vi "Insert Subroutine.vi"(0 "Test Executive in":refnum<class "Test Executive.lvclass">, 1 "Parent ID":string, 5 "Name":string, 9 "File Path":string, 11 "error in (no error)":errorcluster, 12 "Insertion Index":i32=-1, 13 "Path Builder":refnum<class "IPath Builder.lvclass">, 14 "Persistence":refnum<class "IPersist.lvclass">) -> (3 "Unique ID out":string, 4 "Test Executive out":refnum<class "Test Executive.lvclass">, 8 "Replaced?":bool, 15 "error out":errorcluster)   [LabVIEW 2017, in "Test Executive.lvlib" / "Test Executive.lvclass"]
uses:
  <vilib>/gpm_packages/@cs/test-executive/Source/Test Executive/TestExecutive/Test Executive.lvclass
  <vilib>/gpm_packages/@cs/persistence/source/IPersist/IPersist.lvclass
  <vilib>/gpm_packages/@cs/test-executive/Source/Path Builder/IPath Builder/IPath Builder.lvclass
  <vilib>/gpm_packages/@cs/test-executive/Source/Test Executive/Subroutine/Subroutine.lvclass
  <vilib>/gpm_packages/@cs/test-executive/Source/Test Executive/ITestExecutive/ITest Executive.lvclass
  <vilib>/gpm_packages/@cs/test-executive/Source/Test Executive/TestExecutive/Test Executive.lvclass/Test Executive.ctl
  a8f02847-2917-4e0b-9d44-6197dbaaebf7.vi
  ebcf7762-3f7b-48fa-b982-768c2ca258a4.vi
  5e1c43a7-4245-4c3f-80d4-4215ac2c26a8.vi
  5644fd4f-c316-495c-8a03-d45352207638.vi
  1c60c4bb-efd1-4132-9f22-2f49f2b93ccb.vi
  1d71063b-7a03-4771-aede-29323b453e1f.vi
  81d5cec1-e37c-4be8-84f4-52b71e3ef4cd.vi
  972ceb2e-96f1-4f86-b8d7-f01f08263765.vi
  <vilib>/gpm_packages/@cs/linked-list/Source/Linked List/ILinkedList/ILinked List.lvclass
  <vilib>/gpm_packages/@cs/linked-list/Source/Linked List/Linked List Ref/Linked List Ref.lvclass
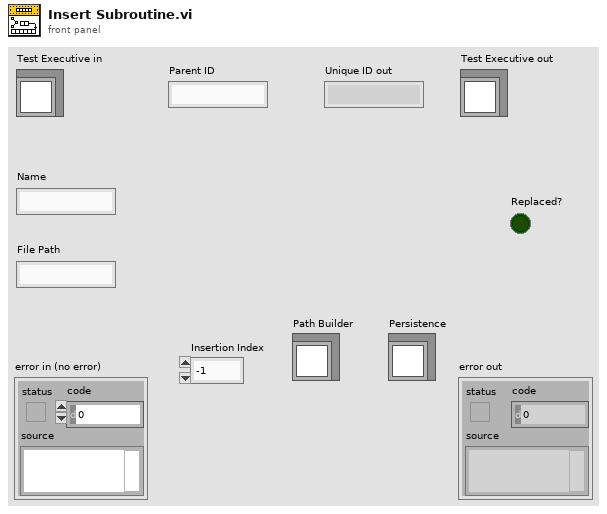
[diagram p1: front panel]
types:
  T1 = enum16{"open", "replace", "create", "open or create", "replace or create", "replace or create with confirmation"}
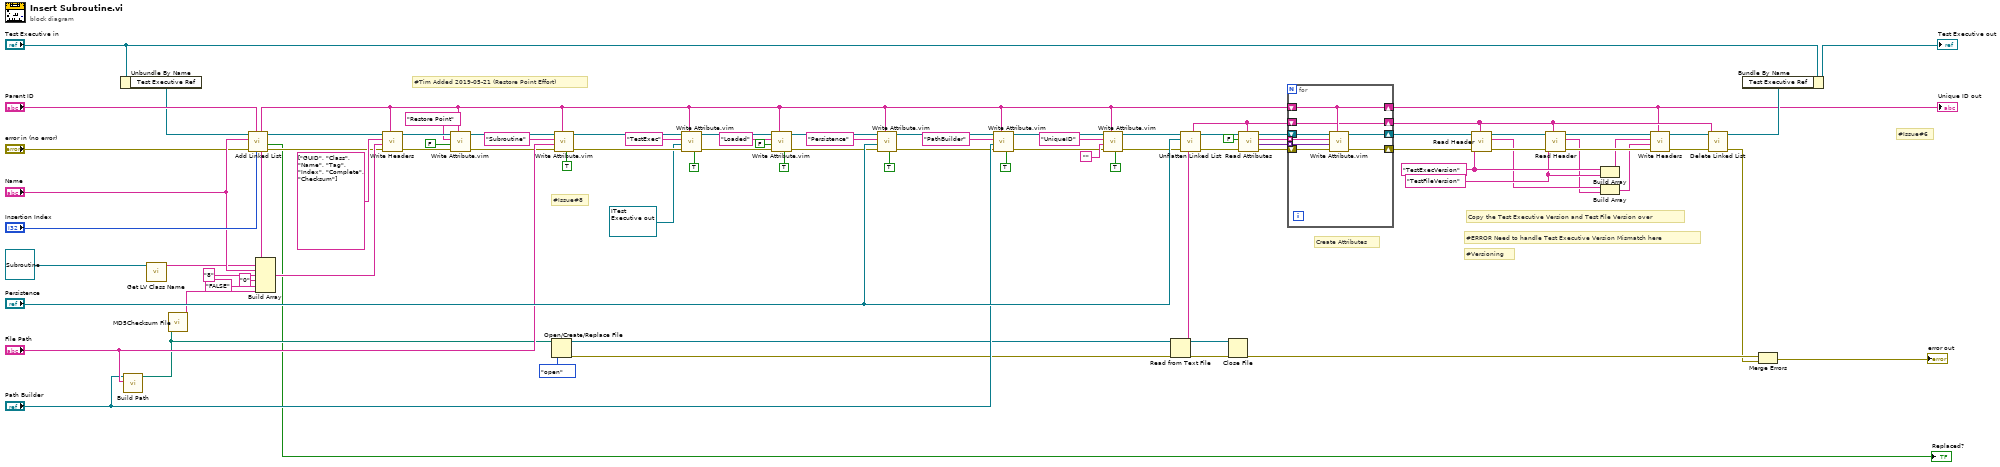
[diagram p0: block diagram]
diagram:
  w7 = "TestFileVersion" ("Header Name")
  w8 = "TestExecVersion" ("Header Name")
  # "#Versioning"
  # "#ERROR Need to handle Test Executive Version Mismatch here"
  # "Copy the Test Executive Version and Test File Version over"
  # "Create Attributes"
  # "#Issue#8"
  # "#Tim Added 2019-05-21 (Restore Point Effort)"
  # "#Issue#6"
  n1 = Unbundle By Name("Test Executive in") -> ("Test Executive Ref"=w27:refnum<data-value>)
  n2 = call-dynamic "Build Path.vi"("Path"="File Path", "IPath Builder in"="Path Builder") -> ("Path"=w26:path)  [unwired: 8 in, 1 out]
  n3 = call <vilib>:"Get LV Class Name.vi"("object"=refnum<class "Subroutine.lvclass"> refnum ("Test Executive.lvlib:Subroutine.lvclass")) -> ("class name"=w75:string)  [unwired: 9 in, 1 out]
  n4 = call <vilib>:"MD5Checksum File.vi"("Path"=w26) -> ("MD5 message-digest"=w61:string)  [unwired: 9 in, 1 out]
  n5 = call <vilib>:"Add Linked List.vi"("Insertion Index"="Insertion Index", "Parent ID"="Parent ID", "error in (no error)"="error in (no error)", "Name"="Name", "Linked List Ref"=w27) -> ("error out"=w76:errorcluster, "Replaced?"=→"Replaced?":bool, "Linked List Ref out"=w77:refnum<data-value>, "Linked List ID out"=w19:string)  [unwired: 3 in]
  n6 = Build Array(w19, w75, "Name", "8" ("Tag"), "0" ("element"), "FALSE" ("element"), w61) -> (w78:string[])
  n7 = call <vilib>:"Write Headers.vi"("Linked List ID"=w19, "error in (no error)"=w76, "Header Values"=w78, "Header Names"=string[] ["GUID", "Class", "Name", "Tag", "Index", "Complete", "Checksum"], "Linked List Ref"=w77) -> ("error out"=w66:errorcluster, "Linked List Ref out"=w67:refnum<data-value>)  [unwired: 5 in]
  n8 = call "Write Attribute.vim"("Linked List ID"=w19, "error in (no error)"=w66, "Attribute"=FALSE, "Attribute Name"="Restore Point", "Linked List Ref"=w67) -> ("error out"=w53:errorcluster, "Linked List Ref out"=w54:refnum<data-value>)  [unwired: 3 in, 2 out]
  n9 = Open/Create/Replace File(file path (use dialog)=w26, operation (0:open)=T1."open") -> (refnum out=w60:refnum<file>, error out=w72:errorcluster)  [unwired: 4 in, 1 out]
  n10 = call "Write Attribute.vim"("Private?"=TRUE, "Linked List ID"=w19, "error in (no error)"=w53, "Attribute"="File Path", "Attribute Name"="Subroutine", "Linked List Ref"=w54) -> ("error out"=w38:errorcluster, "Linked List Ref out"=w40:refnum<data-value>)  [unwired: 2 in, 2 out]
  n11 = call "Write Attribute.vim"("Private?"=TRUE, "Linked List ID"=w19, "error in (no error)"=w38, "Attribute"=refnum<data-value> refnum ("Test Executive Ref out"), "Attribute Name"="TestExec", "Linked List Ref"=w40) -> ("error out"=w37:errorcluster, "Linked List Ref out"=w39:refnum<data-value>)  [unwired: 2 in, 2 out]
  n12 = call "Write Attribute.vim"("Private?"=TRUE, "Linked List ID"=w19, "error in (no error)"=w37, "Attribute"=FALSE, "Attribute Name"="Loaded", "Linked List Ref"=w39) -> ("error out"=w47:errorcluster, "Linked List Ref out"=w48:refnum<data-value>)  [unwired: 2 in, 2 out]
  n13 = call "Write Attribute.vim"("Private?"=TRUE ("Pointer?"), "Linked List ID"=w19, "error in (no error)"=w47, "Attribute"="Persistence", "Attribute Name"="Persistence", "Linked List Ref"=w48) -> ("error out"=w21:errorcluster, "Linked List Ref out"=w23:refnum<data-value>)  [unwired: 2 in, 2 out]
  n14 = call "Write Attribute.vim"("Private?"=TRUE ("Pointer?"), "Linked List ID"=w19, "error in (no error)"=w21, "Attribute"="Path Builder", "Attribute Name"="PathBuilder", "Linked List Ref"=w23) -> ("error out"=w20:errorcluster, "Linked List Ref out"=w22:refnum<data-value>)  [unwired: 2 in, 2 out]
  n15 = call "Write Attribute.vim"("Private?"=TRUE ("Pointer?"), "Linked List ID"=w19, "error in (no error)"=w20, "Attribute"="", "Attribute Name"="UniqueID", "Linked List Ref"=w22) -> ("error out"=w32:errorcluster, "Linked List Ref out"=w33:refnum<data-value>)  [unwired: 2 in, 2 out]
  n16 = Read from Text File(file (use dialog)=w60, error in=w72) -> (refnum out=w71:refnum<file>, text=w69:string, error out=w73:errorcluster)  [unwired: 2 in, 1 out]
  n17 = call <vilib>:"Unflatten Linked List.vi"("Flattened Linked List"=w69, "error in (no error)"=w32, "Persistence"="Persistence", "Linked List Ref"=w33) -> ("error out"=w57:errorcluster, "Linked List Ref out"=w58:refnum<data-value>, "Linked List ID out"=w28:string)  [unwired: 5 in]
  n18 = Close File(refnum=w71, error in=w73) -> (error out=w68:errorcluster)  [unwired: 1 out]
  n19 = call <vilib>:"Read Attributes.vi"("Linked List ID"=w28, "error in (no error)"=w57, "Include Private?"=FALSE, "Linked List Ref"=w58) -> ("error out"=w51:errorcluster, "Attributes"=w1:variant[], "Attribute Names out"=w50:string[], "Linked List Ref out"=w52:refnum<data-value>)  [unwired: 2 in, 2 out]
  n20 = for {
    shift-right: [w97] -> w18
    shift-left: w52 -> [w98]
    shift-right: [w95] -> w17
    shift-left: w51 -> [w96]
    shift-right: [w94] -> w9
    shift-left: w19 -> [w94]
    tunnel: w50 -> [w93] mode=indexing
    shift-right: [w92] -> w16
    shift-left: w28 -> [w92]
    tunnel: w1 -> [w91] mode=indexing
    n21 = call "Write Attribute.vim"("Linked List ID"=w94, "error in (no error)"=w96, "Attribute"=w91, "Attribute Name"=w93, "Linked List Ref"=w98) -> ("error out"=w95:errorcluster, "Linked List Ref out"=w97:refnum<data-value>)  [unwired: 3 in, 2 out]
  }
  "Unique ID out" <- w9
  n22 = call <vilib>:"Read Header.vi"("Linked List ID"=w16, "error in (no error)"=w17, "Header Name"=w8, "Linked List Ref"=w18) -> ("error out"=w14:errorcluster, "Header Value"=w5:string, "Linked List Ref out"=w15:refnum<data-value>)  [unwired: 4 in, 1 out]
  n23 = call <vilib>:"Read Header.vi"("Linked List ID"=w16, "error in (no error)"=w14, "Header Name"=w7, "Linked List Ref"=w15) -> ("error out"=w11:errorcluster, "Header Value"=w4:string, "Linked List Ref out"=w13:refnum<data-value>)  [unwired: 4 in, 1 out]
  n24 = Build Array(w8, w7) -> (w6:string[])
  n25 = Build Array(w5, w4) -> (w3:string[])
  n26 = call <vilib>:"Write Headers.vi"("Linked List ID"=w9, "error in (no error)"=w11, "Header Values"=w3, "Header Names"=w6, "Linked List Ref"=w13) -> ("error out"=w10:errorcluster, "Linked List Ref out"=w12:refnum<data-value>)  [unwired: 5 in]
  n27 = call <vilib>:"Delete Linked List.vi"("error in (no error)"=w10, "Linked List ID"=w16, "Linked List Ref"=w12) -> ("error out"=w29:errorcluster, "Linked List Ref out"=w30:refnum<data-value>)  [unwired: 7 in]
  n28 = Bundle By Name(cluster="Test Executive in", "Test Executive Ref"=w30) -> (→"Test Executive out":refnum<class "Test Executive.lvclass">)
  n29 = Merge Errors(w68, w29) -> (→"error out":errorcluster)
